vi "BigIntMultiply.vi"(1 "b":cluster{"Boolean":bool, "Array":u64[]}, 2 "a":cluster{"Boolean":bool, "Array":u64[]}) -> (0 "a * b":cluster{"Boolean":bool, "Array":u64[]})   [LabVIEW 2023]
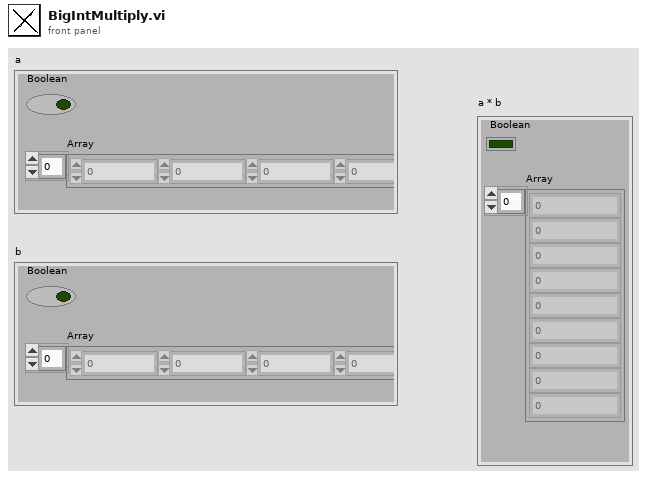
[diagram p1: front panel]
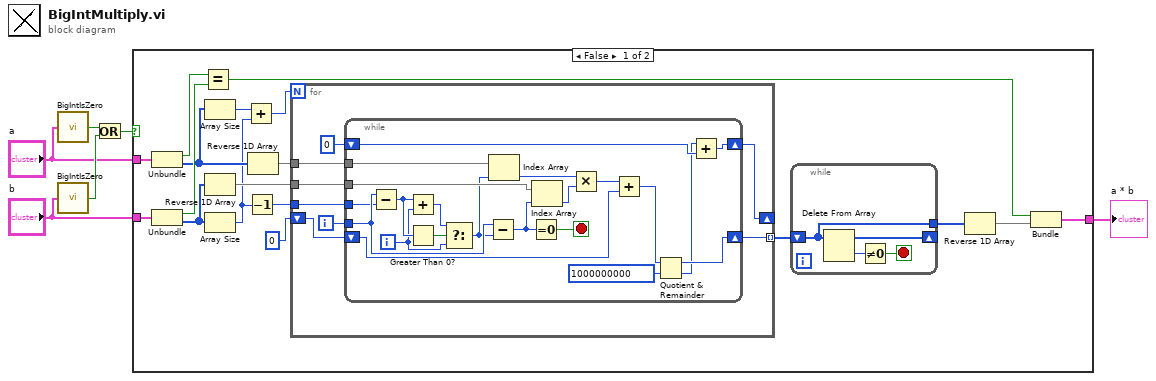
[diagram p0: block diagram]
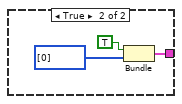
[diagram p2: hidden frame]
diagram:
  n1 = call "BigIntIsZero.vi"("a"="a") -> ("a = 0"=w6:bool)
  n2 = call "BigIntIsZero.vi"("a"="b") -> ("a = 0"=w5:bool)
  n3 = Or(x=w6, y=w5) -> (x .or. y?=w4:bool)
  n4 = case shown="False" w4 {
    tunnel: "a" -> [w24 _]
    tunnel: "b" -> [w23 _]
    tunnel: [w20 w58] -> w1
    frame False {
      n5 = Unbundle(w24) -> ("Boolean"=w22:bool, "Array"=w16:u64[])
      n6 = Unbundle(w23) -> ("Boolean"=w21:bool, "Array"=w15:u64[])
      n7 = Equal?(x=w22, y=w21) -> (x = y?=w19:bool)
      n8 = Array Size(array=w16) -> (size(s)=w17:i32)
      n9 = Reverse 1D Array(array=w15) -> (reversed array=w13:u64[])
      n10 = Array Size(array=w15) -> (size(s)=w8:i32)
      n11 = Add(x=w17, y=w8) -> (x+y=w18:i32)
      n12 = Decrement(x=w8) -> (x-1=w7:i32)
      n13 = Reverse 1D Array(array=w16) -> (reversed array=w14:u64[])
      n14 = for {
        N: w18 -> [_]
        tunnel: w14 -> [w35]
        tunnel: w13 -> [w34]
        tunnel: [w32] -> w10 mode=indexing
        shift-right: [w31] -> _
        shift-left: u64 0 -> [w30]
        tunnel: w7 -> [w29]
        i -> [w36]
        n15 = while {
          tunnel: w36 -> [w43]
          tunnel: w35 -> [w57]
          tunnel: w34 -> [w56]
          shift-right: [w45] -> w32
          shift-left: w30 -> [w52]
          shift-right: [w48] -> w31
          shift-left: u64 0 -> [w49]
          tunnel: w29 -> [w42]
          i -> [w38]
          stop <- w46 stop-if-true
          n16 = Subtract(x=w43, y=w42) -> (x-y=w39:i32)
          n17 = Add(x=w39, y=w38) -> (x+y=w37:i32)
          n18 = Greater Than 0?(x=w39) -> (x > 0?=w40:bool)
          n19 = Select(t=w37, s=w40, f=w38) -> (s? t:f=w41:i32)
          n20 = Subtract(x=w43, y=w41) -> (x-y=w47:i32)
          n21 = Index Array(array=w57, index=w41) -> (element=w55:u64)
          n22 = Equal To 0?(x=w47) -> (x = 0?=w46:bool)
          n23 = Index Array(array=w56, index=w47) -> (element=w54:u64)
          n24 = Multiply(x=w55, y=w54) -> (x*y=w51:u64)
          n25 = Add(x=w51, y=w52) -> (x+y=w50:u64)
          n26 = Quotient & Remainder(x=w50, y=u64 1000000000) -> (x-y*floor(x/y)=w45:u64, floor(x/y)=w44:u64)
          n27 = Add(x=w44, y=w49) -> (x+y=w48:u64)
        }
      }
      n28 = while {
        shift-right: [w26] -> _
        shift-left: w10 -> [w25]
        tunnel: [w25] -> w9
        stop <- w27 stop-if-true
        n29 = Delete From Array(array=w25) -> (deleted portion=w28:u64, array with subset deleted=w26:u64[])  [unwired: 2 in]
        n30 = Not Equal To 0?(x=w28) -> (x != 0?=w27:bool)
      }
      n31 = Reverse 1D Array(array=w9) -> (reversed array=w11:u64[])
      n32 = Bundle(w19, w11) -> (w20:cluster{bool, u64[]})  [unwired: 1 in]
    }
    frame True {
      n33 = Bundle(TRUE, u64[] [0]) -> (w58:cluster{bool, u64[]})  [unwired: 1 in]
    }
  }
  "a * b" <- w1
